vi "FFTimportedtest.vi"() -> ()   [LabVIEW 2015]
doc: "This example shows how to use the FFT functions to interactively filter an image in the frequency domain. First, the Sinusoidal Image Generator VI generates an image with horizontal and vertical sinusoidal patterns. The frequency of these patterns can be controlled from the front panel. \n\nAfter displaying the original image, the VI displays the FFT of the image and then prompts the user to select a region of interest (ROI). If you zoom into the center of the image, or where the high frequency information resides, you will see four dots that represent the +/- vertical and horizontal frequencies. Next, the VI multiplies the mask by the image in the complex domain, and the result is then converted back to the time domain using the IMAQ Inverse FFT function. \n\nNote: To select only the horizontal components of the image, hold down the Ctrl key and select multiple ROIs. This will filter out all of the vertical components."
uses:
  <vilib>/vision/NI_Vision_Development_Module.lvlib
panel:
  in  "Low/High Pass":bool
  in  "Tab Control":T1(tab)
  out "Filtered Image":T2(plugin-control)
  out "Original Image":T2(plugin-control)
  out "FFT Flipped":T2(plugin-control)
  out "FFT":T2(plugin-control)
  out "Mask":T2(plugin-control)
  out "Magnitude Plane":T2(plugin-control)
  # "This program shows how to perform a Mask FFT Filter on an image.\n1) Choose whether you want to perform a Low Pass or High Pass Filter.\n2) Run the VI.\n3) Choose an image from file that you want to perform the masked FFT Fliter on."
  # "High Pass Filter"
  # "Low Pass Filter"
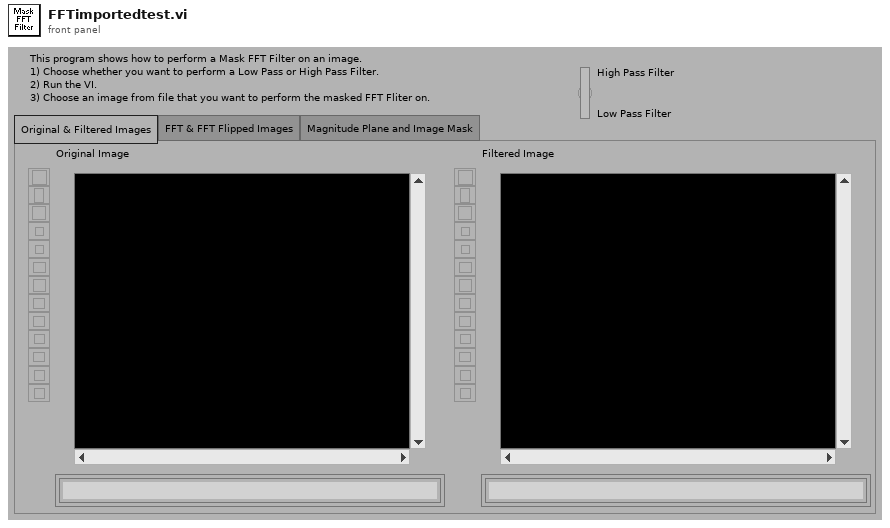
[diagram p1: front panel]
types:
  T1 = enum32{"Original & Filtered Images", "FFT & FFT Flipped Images", "Magnitude Plane and Image Mask"}
  T2 = typedef "IMAQ Image.ctl" = refnum<image>
  T3 = typedef "Image Type" = u32
  T4 = enum32{"Real", "Imaginary", "Magnitude", "Phase"}
  T5 = typedef "ROI Descriptor" = cluster{"Global Rectangle":i32[], "Contours":cluster{"ID":enum32{"External", "Internal"}, "Type":u32, "Coordinates":i32[]}[]}
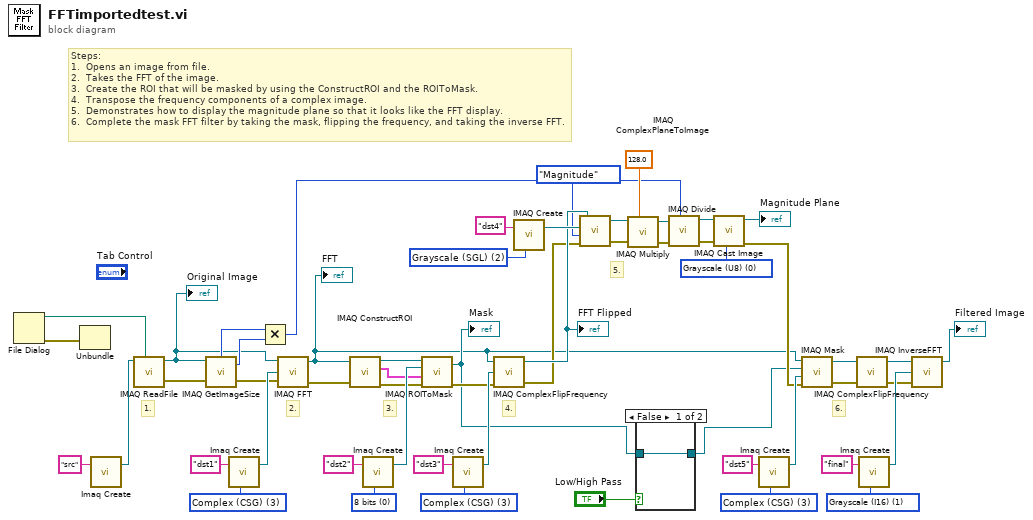
[diagram p0: block diagram]
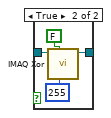
[diagram p2: hidden frame]
diagram:
  w27 = u32 0 items=["8 bits", "16 bits", "Float", "Complex", "RGB", "HSL"] ("Image Type")
  w31 = T3 1 items=["Grayscale (U8)", "Grayscale (I16)", "Grayscale (SGL)", "Complex (CSG)", "RGB (U32)", "HSL (U32)", "RGB (U64)"] ("Image Type")
  w37 = T3 3 items=["Grayscale (U8)", "Grayscale (I16)", "Grayscale (SGL)", "Complex (CSG)", "RGB (U32)", "HSL (U32)", "RGB (U64)"] ("Image Type")
  w38 = T3 0 items=["Grayscale (U8)", "Grayscale (I16)", "Grayscale (SGL)", "Complex (CSG)", "RGB (U32)", "HSL (U32)", "RGB (U64)"] ("Image Type")
  w46 = T3 2 items=["Grayscale (U8)", "Grayscale (I16)", "Grayscale (SGL)", "Complex (CSG)", "RGB (U32)", "HSL (U32)", "RGB (U64)"] ("Image Type")
  w48 = T3 3 items=["Grayscale (U8)", "Grayscale (I16)", "Grayscale (SGL)", "Complex (CSG)", "RGB (U32)", "HSL (U32)", "RGB (U64)"] ("Image Type")
  w51 = T3 3 items=["Grayscale (U8)", "Grayscale (I16)", "Grayscale (SGL)", "Complex (CSG)", "RGB (U32)", "HSL (U32)", "RGB (U64)"] ("Image Type")
  # "4."
  # "6."
  # "5."
  # "3."
  # "2."
  # "1."
  # "Steps:\n1.  Opens an image from file.\n2.  Takes the FFT of the image.\n3.  Create the ROI that will be masked by using the ConstructROI and the ROIToMask.\n4.  Transpose the frequency components of a complex image.\n5.  Demonstrates how to display the magnitude plane so that it looks like the FFT display.\n6.  Complete the mask FFT filter by taking the mask, flipping the frequency, and taking the inverse FFT."
  n1 = File Dialog() -> (0:w3:errorcluster, 3:w53:path)  [unwired: 7 in, 2 out]
  n2 = Unbundle(w3) -> ()  [unwired: 3 out]
  n3 = call "Imaq Create"("Image Name"="src") -> ("New Image"=w54:T2)  [unwired: 4 in, 1 out]
  n4 = call "IMAQ ReadFile"("File Path"=w53, "Image"=w54) -> ("error out"=w13:errorcluster, "Image Out"=w10:T2)  [unwired: 5 in, 3 out]
  "Original Image" <- w10
  n5 = call "IMAQ GetImageSize"("Image"=w10, "error in (no error)"=w13) -> ("Y Resolution"=w28:i32, "X Resolution"=w11:i32, "error out"=w12:errorcluster)  [unwired: 2 in]
  n6 = call "Imaq Create"("Image Name"="dst1", "Image Type"=w51) -> ("New Image"=w50:T2)  [unwired: 3 in, 1 out]
  n7 = Multiply(x=w11, y=w28) -> (x*y=w14:i32)
  n8 = call "IMAQ FFT"("error in (no error)"=w12, "Image Dst"=w50, "Image Src"=w10) -> ("error out"=w22:errorcluster, "Image Dst Out"=w1:T2)  [unwired: 1 in]
  "FFT" <- w1
  n9 = call "IMAQ ConstructROI"("error in (no error)"=w22, "Image"=w1) -> ("error out"=w21:errorcluster, "ROI Descriptor Out"=w4:T5, "Image Out (duplicate)"=w25:T2)  [unwired: 6 in, 1 out]
  n10 = call "Imaq Create"("Image Name"="dst2", "Image Type"=w27) -> ("New Image"=w26:T2)  [unwired: 3 in, 1 out]
  n11 = call "IMAQ ROIToMask"("error in (no error)"=w21, "ROI Descriptor"=w4, "Image"=w26, "Image Model"=w25) -> ("error out"=w20:errorcluster, "Image Out"=w6:T2)  [unwired: 2 in, 1 out]
  "Mask" <- w6
  n12 = call "Imaq Create"("Image Name"="dst3", "Image Type"=w48) -> ("New Image"=w47:T2)  [unwired: 3 in, 1 out]
  n13 = call "IMAQ ComplexFlipFrequency"("error in (no error)"=w20, "Image Dst"=w47, "Image Src"=w1) -> ("error out"=w8:errorcluster, "Image Dst Out"=w15:T2)  [unwired: 1 in]
  "FFT Flipped" <- w15
  n14 = call "IMAQ Create"("Image Name"="dst4", "Image Type"=w46) -> ("New Image"=w44:T2)  [unwired: 3 in, 1 out]
  n15 = call "IMAQ ComplexPlaneToImage"("error in (no error)"=w8, "Plane"=T4."Magnitude", "Image Dst"=w44, "Image Src"=w15) -> ("error out"=w18:errorcluster, "Image Dst Out"=w43:T2)  [unwired: 1 in]
  n16 = call "IMAQ Multiply"("Image Src A"=w43, "Constant"=sgl 128.0, "error in (no error)"=w18) -> ("Image Dst Out"=w41:T2, "error out"=w17:errorcluster)  [unwired: 4 in]
  n17 = case shown="False" "Low/High Pass" {
    tunnel: [w56 w58] -> w5
    tunnel: w6 -> [w56 w57]
    frame False {
    }
    frame True {
      n18 = call "IMAQ Xor"("Constant"=255, "Xor/Xnor (Xor)"=FALSE ("And/Nand (And)"), "Image Src A"=w57) -> ("Image Dst Out"=w58:T2)  [unwired: 7 in, 1 out]
    }
  }
  n19 = call "IMAQ Divide"("Image Src A"=w41, "Constant"=w14, "error in (no error)"=w17) -> ("Image Dst Out"=w39:T2, "error out"=w16:errorcluster)  [unwired: 4 in]
  n20 = call "IMAQ Cast Image"("Image Type"=w38, "error in (no error)"=w16, "Image Src"=w39) -> ("error out"=w7:errorcluster, "Image Dst Out"=→"Magnitude Plane":T2)  [unwired: 7 in]
  n21 = call "Imaq Create"("Image Name"="dst5", "Image Type"=w37) -> ("New Image"=w36:T2)  [unwired: 3 in, 1 out]
  n22 = call "IMAQ Mask"("error in (no error)"=w7, "Image Dst"=w36, "Image Mask"=w5, "Image Src"=w1) -> ("error out"=w23:errorcluster, "Image Dst Out"=w34:T2)  [unwired: 1 in]
  n23 = call "IMAQ ComplexFlipFrequency"("error in (no error)"=w23, "Image Src"=w34) -> ("error out"=w19:errorcluster, "Image Dst Out"=w33:T2)  [unwired: 2 in]
  n24 = call "Imaq Create"("Image Name"="final", "Image Type"=w31) -> ("New Image"=w29:T2)  [unwired: 3 in, 1 out]
  n25 = call "IMAQ InverseFFT"("error in (no error)"=w19, "Image Dst"=w29, "Image Src"=w33) -> ("Image Dst Out"=→"Filtered Image":T2)  [unwired: 1 in, 1 out]
